vi "FGV CAN Daten.vi"(6 "Aktionen":T6, 8 "Status":u32[](array[numeric]), 9 "data":T3=[{"timestamp"=timestamp(0 s since 1904-01-01), "payload"=[0, 2, 3, 4, 5, 6, 7, 8], "identifier"=2, "type"=0, "extended?"=FALSE, "echo?"=FALSE}, {"timestamp"=timestamp(0 s since 1904-01-01), "payload"=[0, 1, 2, 3, 4, 5, 6, 7], "identifier"=3, "type"=0, "extended?"=FALSE, "echo?"=FALSE}] {"payload" format="%x"; "timestamp" format="%<%.7X\n%x>T"; "type" items=["CAN Data"=0, "CAN Remote"=1, "CAN Bus Error"=2, "CAN 2.0 Data"=8, "CAN FD Data"=16, "CAN FD+BRS Data"=24, "J1939 Data"=192, "Delay"=224, "Log Trigger"=225, "Start Trigger"=226]; "identifier" format="%x"}, 11 "Konfig Daten 2":T1={"Baude Rate"=250000, "COM state"=144, "Frame-ID FTIR Start"=0, "Frame-ID FTIR End"=0, "Frame-ID Status Start"=0, "Frame-ID Status End"=0, "Zustand Information"=0, "Aktion"=0, "Frame-ID FTIR Arry"=[], "Frame-ID Status Arry"=[], "GPS Start"=0, "Interface"="CAN1"} {"Baude Rate" items=["40 kBaud"=40000, "50 kBaud"=50000, "62,5 kBaud"=62500, "80 kBaud"=80000, "83,3 kBaud"=83300, "100 kBaud"=100000, "125 kBaud"=125000, "160 kBaud"=160000, "200 kBaud"=200000, "250 kBaud"=250000, "400 kBaud"=400000, "500 kBaud"=500000, "800 kBaud"=800000, "1 MBaud"=1000000]}) -> (0 "Status":u32[](array[numeric]), 1 "data":T4[](array[typedef])=[{"timestamp"=timestamp(0 s since 1904-01-01), "payload"=[0, 2, 3, 4, 5, 6, 7, 8], "identifier"=2, "type"=0, "extended?"=FALSE, "echo?"=FALSE}, {"timestamp"=timestamp(0 s since 1904-01-01), "payload"=[0, 1, 2, 3, 4, 5, 6, 7], "identifier"=3, "type"=0, "extended?"=FALSE, "echo?"=FALSE}] {"payload" format="%x"; "timestamp" format="%<%.7X\n%x>T"; "type" items=["CAN Data"=0, "CAN Remote"=1, "CAN Bus Error"=2, "CAN 2.0 Data"=8, "CAN FD Data"=16, "CAN FD+BRS Data"=24, "J1939 Data"=192, "Delay"=224, "Log Trigger"=225, "Start Trigger"=226]; "identifier" format="%x"}, 3 "Konfig Daten":T1={"Baude Rate"=250000, "COM state"=144, "Frame-ID FTIR Start"=0, "Frame-ID FTIR End"=0, "Frame-ID Status Start"=0, "Frame-ID Status End"=0, "Zustand Information"=0, "Aktion"=0, "Frame-ID FTIR Arry"=[], "Frame-ID Status Arry"=[], "GPS Start"=0, "Interface"="CAN1"} {"Baude Rate" items=["40 kBaud"=40000, "50 kBaud"=50000, "62,5 kBaud"=62500, "80 kBaud"=80000, "83,3 kBaud"=83300, "100 kBaud"=100000, "125 kBaud"=125000, "160 kBaud"=160000, "200 kBaud"=200000, "250 kBaud"=250000, "400 kBaud"=400000, "500 kBaud"=500000, "800 kBaud"=800000, "1 MBaud"=1000000]})   [LabVIEW 2020, in "CAN Interface.lvlib"]
uses:
  CAN Interface.lvlib
  <vilib>/xnet/xnet.llb/XNET Frame CAN.ctl
  <vilib>/xnet/xnet.llb/XNET Frame Type CAN.ctl
  FGV CAN Daten Aktionen.ctl
  CAN Data.ctl
  Seiten/CAN Konfig/Konfig Daten PC.ctl
  Baude Rate.ctl
  Seiten/CAN Konfig/CAN Konfig.lvlib
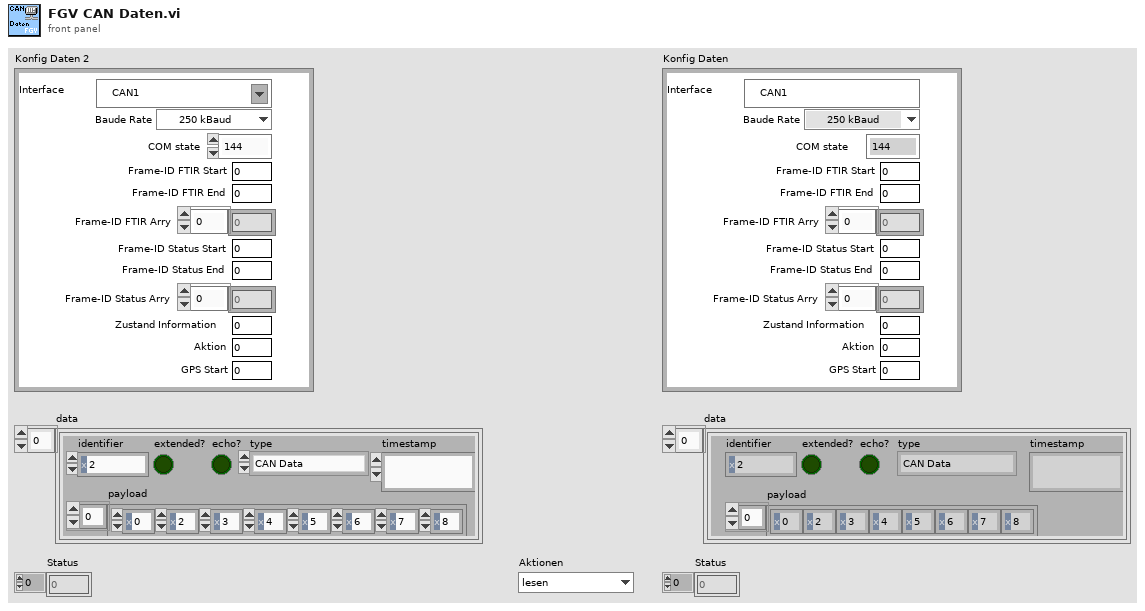
[diagram p1: front panel]
types:
  T1 = typedef "CAN Konfig.lvlib/Konfig Daten PC.ctl" = cluster{"Baude Rate":T2, "COM state":u8, "Frame-ID FTIR Start":u32, "Frame-ID FTIR End":u32, "Frame-ID Status Start":u32, "Frame-ID Status End":u32, "Zustand Information":u32, "Aktion":u32, "Frame-ID FTIR Arry":u32[], "Frame-ID Status Arry":u32[], "GPS Start":u32, "Interface":refnum<k21>}
  T2 = typedef "CAN Interface.lvlib/Baude Rate.ctl" = u32
  T3 = typedef "CAN Interface.lvlib/CAN Data.ctl" = T4[]
  T4 = typedef "XNET Frame CAN.ctl" = cluster{"timestamp":timestamp, "payload":u8[], "identifier":u32, "type":T5, "extended?":bool, "echo?":bool}
  T5 = typedef "XNET Frame Type CAN.ctl" = u8
  T6 = typedef "CAN Interface.lvlib/FGV CAN Daten Aktionen.ctl" = enum16{"lesen", "Daten", "Konfig", "laden", "speichern", "Status"}
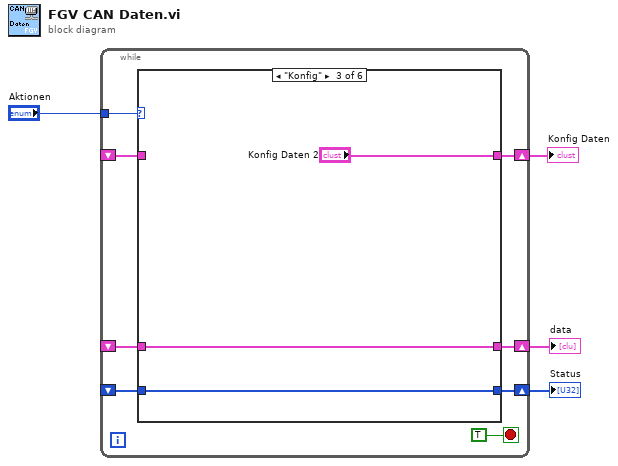
[diagram p0: block diagram]
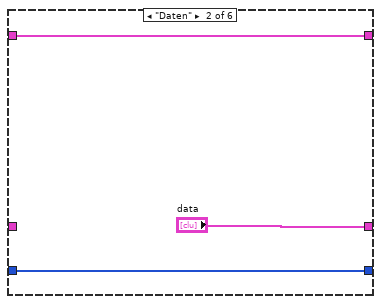
[diagram p3: hidden frame]
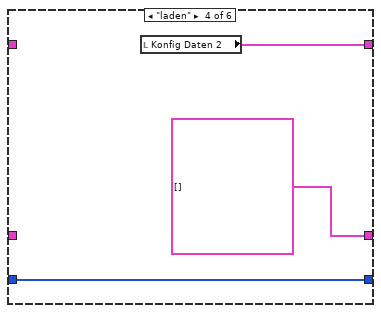
[diagram p4: hidden frame]
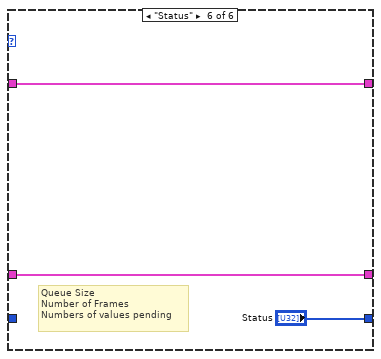
[diagram p6: hidden frame]
diagram:
  n1 = while {
    tunnel: "Aktionen" -> [w11]
    shift-right: [w10] -> w3
    shift-left: _ -> [w9]
    shift-right: [w8] -> w1
    shift-left: _ -> [w7]
    shift-right: [w6] -> w2
    shift-left: _ -> [w5]
    stop <- TRUE stop-if-true
    n2 = case shown="\"Konfig\"" w11 {
      tunnel: [w15 "data" w21 T4[] [] ("data") w26 w30] -> w10
      tunnel: w9 -> [w15 _ w21 _ w26 w30]
      tunnel: [w14 w18 "Konfig Daten 2" w22 w27 w29] -> w8
      tunnel: w7 -> [w14 w18 _ _ w27 w29]
      tunnel: [w13 w17 w20 w23 w25 "Status"] -> w6
      tunnel: w5 -> [w13 w17 w20 w23 w25 _]
      frame "lesen", Default {
      }
      frame "Daten" {
      }
      frame "Konfig" {
      }
      frame "laden" {
        n3 = local read "Konfig Daten 2"() -> (w22:T1)
      }
      frame "speichern" {
      }
      frame "Status" {
        # "Queue Size\nNumber of Frames\nNumbers of values pending"
      }
    }
  }
  "data" <- w3
  "Status" <- w2
  "Konfig Daten" <- w1
